vi "Scale Deadzone.vi"(9 "deadzone":i32=10240, 10 "scaling factor":i32=88, 11 "input value":i32) -> (2 "output value":i32)   [LabVIEW 2009]
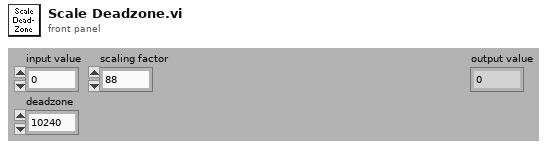
[diagram p1: front panel]
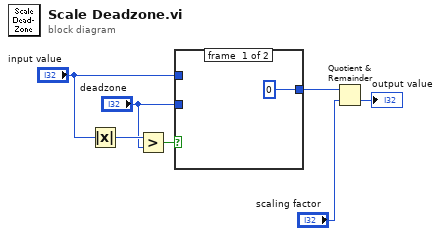
[diagram p0: block diagram]
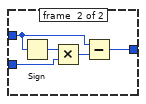
[diagram p2: hidden frame]
diagram:
  n1 = Absolute Value(x="input value") -> (abs(x)=w6:i32)
  n2 = Greater?(x=w6, y="deadzone") -> (0:w7:bool)
  n3 = case shown="True" w7 {
    tunnel: [0 w13] -> w5
    tunnel: "input value" -> [_ w12]
    tunnel: "deadzone" -> [_ w9]
    frame #0 {
    }
    frame #1 {
      n4 = Sign(1:w12) -> (0:w10:i32)
      n5 = Multiply(x=w10, y=w9) -> (x*y=w11:i32)
      n6 = Subtract(x=w12, y=w11) -> (x-y=w13:i32)
    }
  }
  n7 = Quotient & Remainder(x=w5, y="scaling factor") -> (floor(x/y)=→"output value":i32)  [unwired: 1 out]
